vi "Flush All FIFOs.vi"(8 "Error In":errorcluster, 11 "FPGA Ref":T1) -> (0 "Error Out":errorcluster)   [LabVIEW 2020]
doc: "Stops the acquisition."
uses:
  RIG-SPECIFIC FILES/FPGA Refs/FPGA Ref.ctl
  Global Variables/General Globals.vi
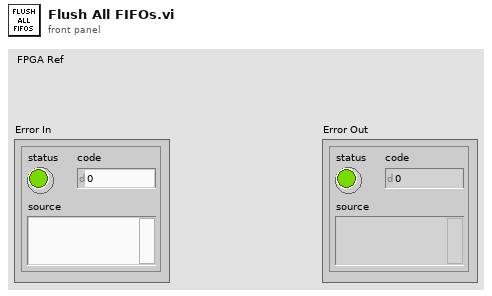
[diagram p1: front panel]
types:
  T1 = typedef "FPGA Ref.ctl" = refnum<k20>
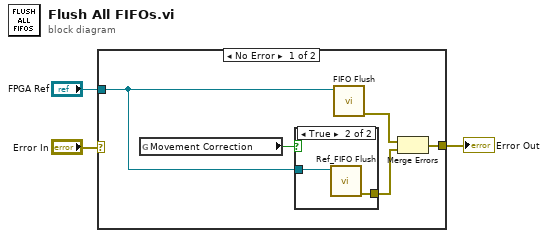
[diagram p0: block diagram]
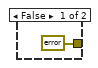
[diagram p2: hidden frame]
diagram:
  n1 = case shown="No Error" "Error In" {
    selector: "Error In" -> [_ w12]
    tunnel: [w8 w12] -> w2
    tunnel: "FPGA Ref" -> [w4 _]
    frame No Error {
      n2 = global read "General Globals.vi" "Movement Correction"() -> (w7:bool)
      n3 = case shown="True" w7 {
        tunnel: w4 -> [_ w10]
        tunnel: [errorcluster {"status"=FALSE, "code"=0, "source"=""} ("Error Out") w11] -> w6
        frame False {
        }
        frame True {
          n4 = call "Ref_FIFO Flush.vi"("FPGA VI Ref"=w10) -> ("Error Out"=w11:errorcluster)  [unwired: 9 in, 1 out]
        }
      }
      n5 = call "FIFO Flush.vi"("FPGA VI Ref"=w4) -> ("Error Out"=w5:errorcluster)  [unwired: 8 in, 2 out]
      n6 = Merge Errors(w5, w6) -> (w8:errorcluster)
    }
    frame Error {
    }
  }
  "Error Out" <- w2
